vi "Arduino_Compile.vi"(8 "error in (no error)":errorcluster, 10 "Code":string="/*\n  Blink\n\n  Turns an LED on for one second, then off for one second, repeatedly.\n\n  Most Arduinos have an on-board LED you can control. On the UNO, MEGA and ZERO\n  it is attached to digital pin 13, on MKR1000 on pin 6. LED_BUILTIN is set to\n  the correct LED pin independent of which board is used.\n  If you want to know what pin the on-board LED is connected to on your Arduino\n  model, check the Technical Specs of your board at:\n  https://www.arduino.cc/en/Main/Products\n\n  modified 8 May 2014\n  by Scott Fitzgerald\n  modified 2 Sep 2016\n  by Arturo Guadalupi\n  modified 8 Sep 2016\n  by Colby Newman\n\n  This example code is in the public domain.\n\n  http://www.arduino.cc/en/Tutorial/Blink\n*/\n\n// the setup function runs once when you press reset or power the board\nvoid setup() {\n  // initialize digital pin LED_BUILTIN as an output.\n  pinMode(LED_BUILTIN, OUTPUT);\n}\n\n// the loop function runs over and over again forever\nvoid loop() {\n  digitalWrite(LED_BUILTIN, HIGH);   // turn the LED on (HIGH is the voltage level)\n  delay(1000);                       // wait for a second\n  digitalWrite(LED_BUILTIN, LOW);    // turn the LED off by making the voltage LOW\n  delay(1000);                       // wait for a second\n}", 11 "Board":string="Arduino Nano 33 IoT") -> (0 "error out":errorcluster, 3 "Arduino Out":T1={"Java"=path "/Applications/Arduino.app/Contents/Java", "Packages"=path "/Users/crogers/Library/Arduino15/packages", "folder"=path "/Users/crogers/Documents/LabVIEW Data", "serial"="/dev/cu.usbmodem14301", "Console"="***** Complie *****\nSketch uses 11292 bytes (4%) of program storage space. Maximum is 262144 bytes.\n\n\n"})   [LabVIEW 2022 SP3]
uses:
  Arduino.ctl
panel:
  out "Console":string="/*\n  Blink\n\n  Turns an LED on for one second, then off for one second, repeatedly.\n\n  Most Arduinos have an on-board LED you can control. On the UNO, MEGA and ZERO\n  it is attached to digital pin 13, on MKR1000 on pin 6. LED_BUILTIN is set to\n  the correct LED pin independent of which board is used.\n  If you want to know what pin the on-board LED is connected to on your Arduino\n  model, check the Technical Specs of your board at:\n  https://www.arduino.cc/en/Main/Products\n\n  modified 8 May 2014\n  by Scott Fitzgerald\n  modified 2 Sep 2016\n  by Arturo Guadalupi\n  modified 8 Sep 2016\n  by Colby Newman\n\n  This example code is in the public domain.\n\n  http://www.arduino.cc/en/Tutorial/Blink\n*/\n\n// the setup function runs once when you press reset or power the board\nvoid setup() {\n  // initialize digital pin LED_BUILTIN as an output.\n  pinMode(LED_BUILTIN, OUTPUT);\n}\n\n// the loop function runs over and over again forever\nvoid loop() {\n  digitalWrite(LED_BUILTIN, HIGH);   // turn the LED on (HIGH is the voltage level)\n  delay(1000);                       // wait for a second\n  digitalWrite(LED_BUILTIN, LOW);    // turn the LED off by making the voltage LOW\n  delay(1000);                       // wait for a second\n}"
  in  "Arduino In":T1={"Java"=path "/Applications/Arduino.app/Contents/Java", "Packages"=path "/Users/crogers/Library/Arduino15/packages", "folder"=path "", "serial"="", "Console"=""}
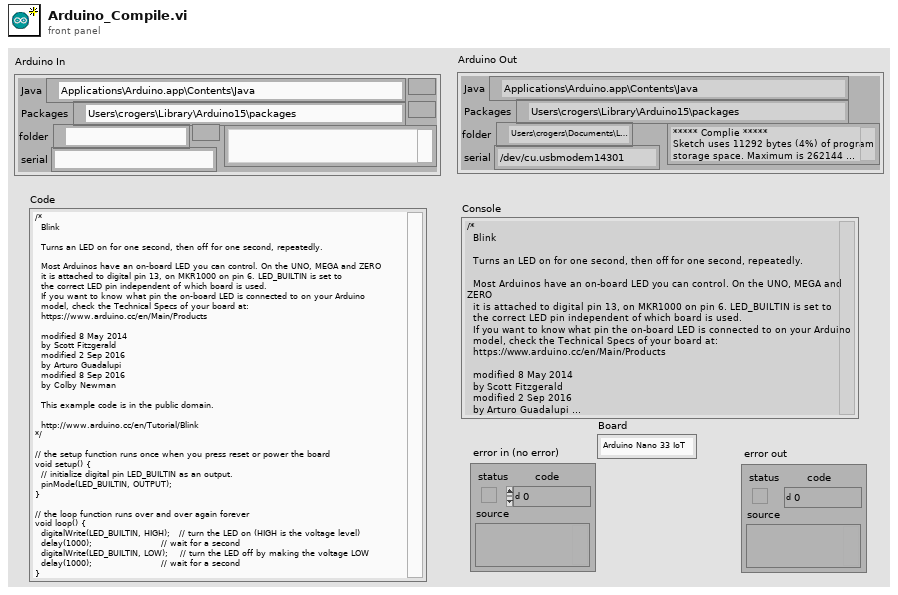
[diagram p1: front panel]
types:
  T1 = typedef "Arduino.ctl" = cluster{"Java":path, "Packages":path, "folder":path, "serial":string, "Console":string}
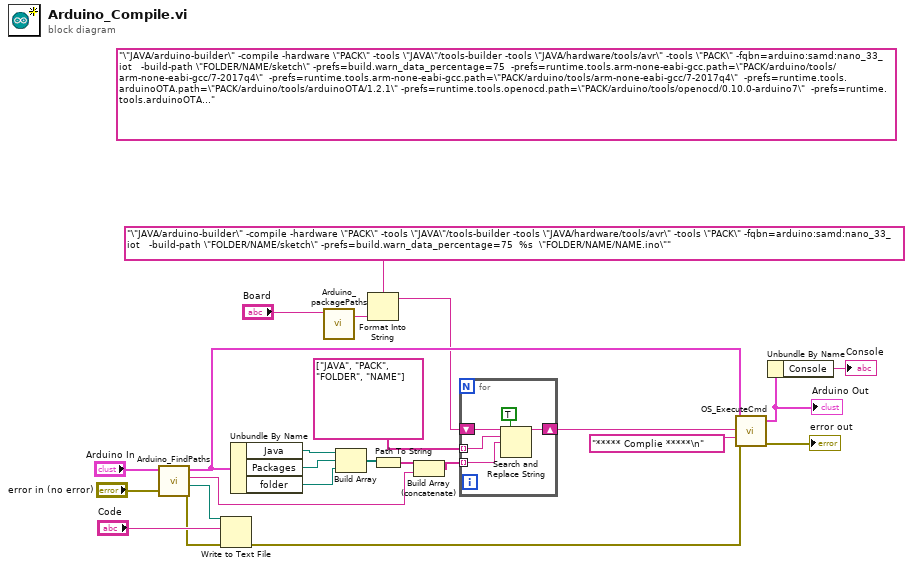
[diagram p0: block diagram]
diagram:
  (unwired) "\"JAVA/arduino-builder\" -compile -hardware \"PACK\" -tools \"JAVA\"/tools-builder -tools \"JAVA/hardware/tools/avr\" -tools \"PACK\" -fqbn=arduino:samd:nano_33_iot   -build-path \"FOLDER/NAME/sketch\" -prefs=build.warn_data_percentage=75  -prefs=runtime.tools.arm-none-eabi-gcc.path=\"PACK/arduino/tools/arm-none-eabi-gcc/7-2017q4\"  -prefs=runtime.tools.arm-none-eabi-gcc.path=\"PACK/arduino/tools/arm-none-eabi-gcc/7-2017q4\"  -prefs=runtime.tools.arduinoOTA.path=\"PACK/arduino/tools/arduinoOTA/1.2.1\" -prefs=runtime.tools.openocd.path=\"PACK/arduino/tools/openocd/0.10.0-arduino7\"  -prefs=runtime.tools.arduinoOTA-1.2.1.path=\"PACK/arduino/tools/arduinoOTA/1.2.1\" -prefs=runtime.tools.openocd-0.10.0-arduino7.path=\"PACK/arduino/tools/openocd/0.10.0-arduino7\" \"FOLDER/NAME/NAME.ino\"" ("string")
  n1 = call "Arduino_FindPaths.vi"("error in (no error)"="error in (no error)", "Arduino In"="Arduino In") -> ("error out"=w7:errorcluster, "temp code file"=w5:path, "Name"=w6:string, "Arduino In out"=w11:T1)  [unwired: 6 in]
  n2 = Write to Text File(file (use dialog)=w5, text="Code", error in=w7) -> (error out=w24:errorcluster)  [unwired: 1 in, 2 out]
  n3 = Unbundle By Name(w11) -> ("Java"=w15:path, "Packages"=w14:path, "folder"=w9:path)
  n4 = call "Arduino_packagePaths.vi"("name"="Board") -> ("String"=w3:string)  [unwired: 10 in]
  n5 = Build Array(w15, w14, w9) -> (w18:path[])
  n6 = Format Into String(format string="\"JAVA/arduino-builder\" -compile -hardware \"PACK\" -tools \"JAVA\"/tools-builder -tools \"JAVA/hardware/tools/avr\" -tools \"PACK\" -fqbn=arduino:samd:nano_33_iot   -build-path \"FOLDER/NAME/sketch\" -prefs=build.warn_data_percentage=75  %s  \"FOLDER/NAME/NAME.ino\"" ("string"), w3) -> (resulting string=w2:string)  [unwired: 2 in, 1 out]
  n7 = Path To String(path=w18) -> (string=w17:string[])
  n8 = Build Array (concatenate)(w17, w6) -> (w16:string[])
  n9 = for {
    shift-right: [w27] -> w22
    shift-left: w2 -> [w28]
    tunnel: string[] ["JAVA", "PACK", "FOLDER", "NAME"] -> [w26] mode=indexing
    tunnel: w16 -> [w25] mode=indexing
    n10 = Search and Replace String(replace all?=TRUE ("replace all? (F)"), input string=w28, search string=w26, replace string=w25) -> (result string=w27:string)  [unwired: 4 in, 3 out]
  }
  n11 = call "OS_ExecuteCmd.vi"("error in (no error)"=w24, "Comment"="***** Complie *****\n" ("string"), "Command"=w22, "Arduino In"=w11) -> ("error out"=→"error out":errorcluster, "Arduino out"=w13:T1)  [unwired: 6 in]
  "Arduino Out" <- w13
  n12 = Unbundle By Name(w13) -> ("Console"=→"Console":string)
